vi "FTW-Endpoint-TCP-Reply-Send-Worker.vi"(0 "TCP Endpoint":refnum<class "FTW-Endpoint-TCP.lvclass">) -> ()   [LabVIEW 2013, in "FTW-Endpoint-TCP.lvclass"]
uses:
  FTW-Endpoint-TCP.lvclass
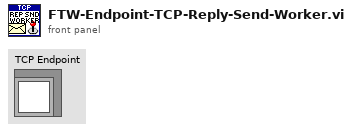
[diagram p1: front panel]
types:
  T1 = typedef "FTW-MessagePayload.ctl" = cluster{"Header":string, "Body":string, "FTW: Sender Identity":string, "FTW: Reply Address":string, "FTW: Reply Error":errorcluster}
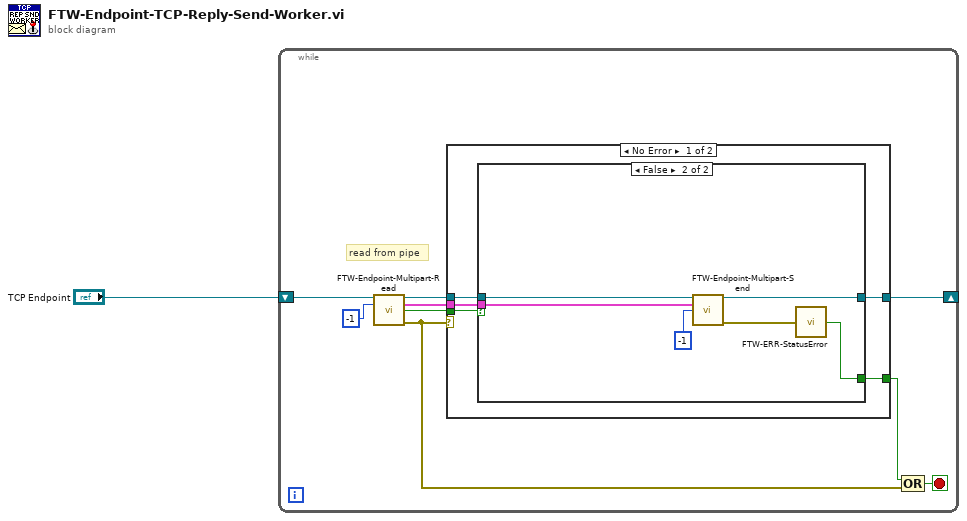
[diagram p0: block diagram]
diagram:
  n1 = while {
    shift-right: [w10] -> _
    shift-left: "TCP Endpoint" -> [w9]
    stop <- w8 stop-if-true
    # "read from pipe"
    n2 = call-dynamic "FTW-Endpoint-Multipart-Read.vi"("FTW Endpoint"=w9, "Timeout"=-1) -> ("FTW Endpoint out"=w6:refnum<class "FTW-Endpoint-TCP.lvclass">, "Message Received"=w4:T1, "Timed out?"=w5:bool, "error out"=w7:errorcluster)  [unwired: 10 in]
    n3 = case shown="No Error" w7 {
      tunnel: [w15 w23] -> w10
      tunnel: w6 -> [w14 w23]
      tunnel: w5 -> [w13 _]
      tunnel: w4 -> [w12 _]
      tunnel: [w11 _] -> w3
      frame No Error {
        n4 = case shown="False" w13 {
          tunnel: w14 -> [w16 w22]
          tunnel: [w16 w21] -> w15
          tunnel: [_ w19] -> w11
          tunnel: w12 -> [_ w17]
          frame True {
            # "timeout\ndo nothing"
          }
          frame False {
            n5 = call-dynamic "FTW-Endpoint-Multipart-Send.vi"("FTW Endpoint"=w22, "Message"=w17, "Timeout"=-1) -> ("FTW Endpoint out"=w21:refnum<class "FTW-Endpoint-TCP.lvclass">, "error out"=w20:errorcluster)  [unwired: 10 in, 1 out]
            n6 = call "FTW-ERR-StatusError.vi"("error to check"=w20) -> ("Error?"=w19:bool)
          }
        }
      }
      frame Error {
      }
    }
    n7 = Compound Arithmetic op=OR(w3, w7) -> (w8:bool)
  }
